vi "PXI M-Series Sync.vi"() -> ()   [LabVIEW 2012]
uses:
  <vilib>/DAQmx/write.llb/DAQmx Write (Analog 2D DBL NChan NSamp).vi
  <vilib>/DAQmx/read.llb/DAQmx Read (Digital 1D U32 1Chan NSamp).vi
  <vilib>/DAQmx/read.llb/DAQmx Read (Analog 2D I16 NChan NSamp).vi
  <vilib>/DAQmx/create/channels.llb/DAQmx Create Channel (AI-Voltage-Basic).vi
  <vilib>/DAQmx/configure/timing.llb/DAQmx Timing (Sample Clock).vi
  <vilib>/DAQmx/create/channels.llb/DAQmx Create Channel (AO-Voltage-Basic).vi
  <vilib>/DAQmx/create/channels.llb/DAQmx Create Channel (DI-Digital Input).vi
  <vilib>/DAQmx/miscellaneous.llb/DAQmx Fill In Error Info.vi
  <resource>/objmgr/daqmx.rc
panel:
  out "Trig2":bool
  out "Trig1":bool
  out "Alternative predicted rate AO":dbl
  out "RefClk.Rate":dbl
  out "SampClk.TimebaseDiv":u32
  out "SampClk.MaxRate":dbl
  in  "Desired sample rate":dbl=200000.0
  out "Predicted sample rate AI":dbl
  out "Real sample rate AI":dbl
  out "AI.Rng.Low":dbl
  out "AI.Rng.High":dbl
  out "AvailSampPerChan":u32
  out "Analog in":i16[][](graph)
  in  "stop":bool
  out "error out":errorcluster
  # "AI"
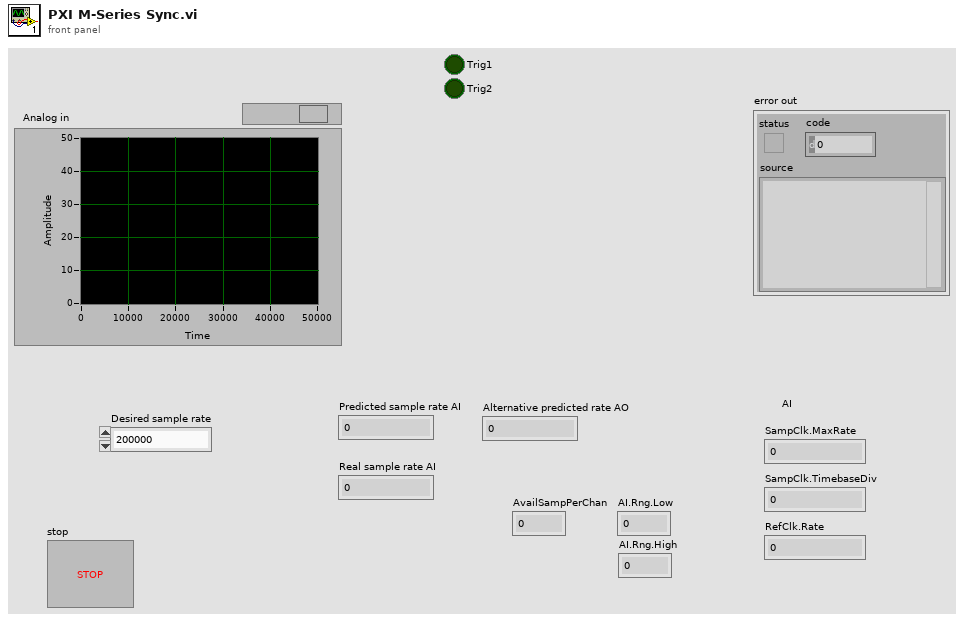
[diagram p1: front panel]
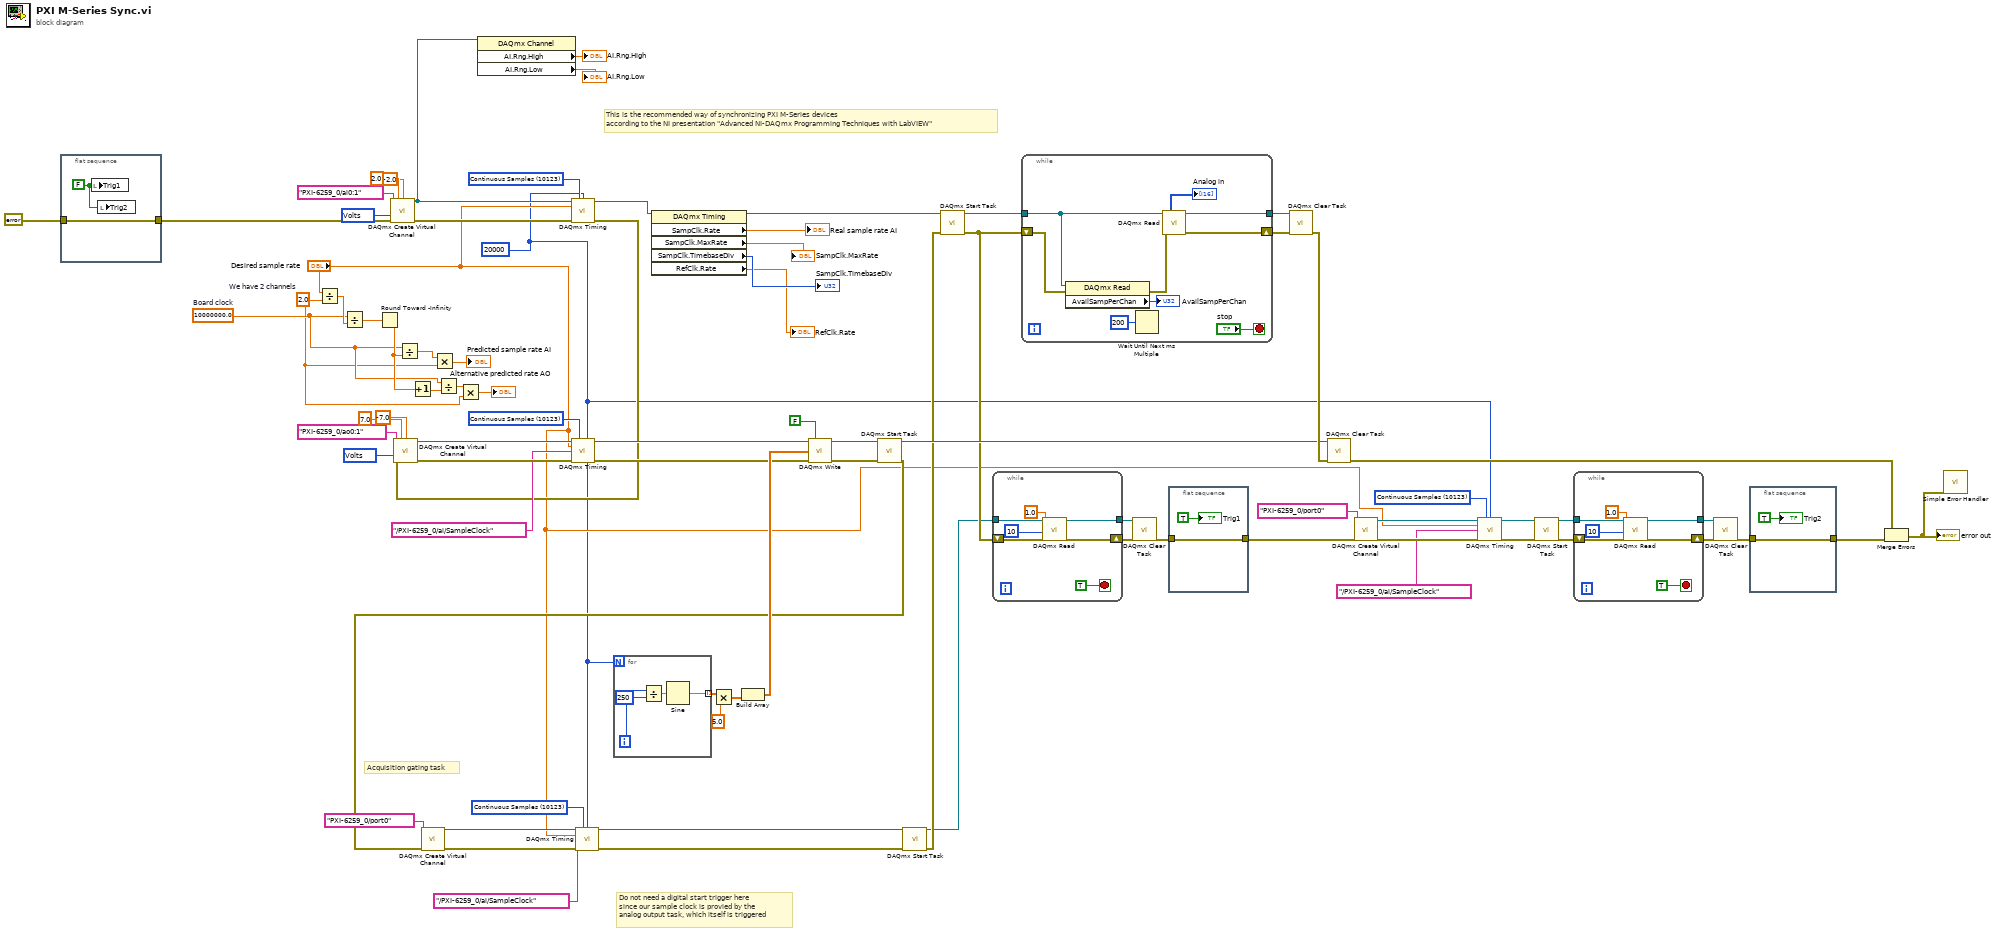
[diagram p0: block diagram]
diagram:
  w13 = 10123 items=["Finite Samples"=10178, "Continuous Samples"=10123, "Hardware Timed Single Point"=12522] ("sample mode")
  w36 = 10123 items=["Finite Samples"=10178, "Continuous Samples"=10123, "Hardware Timed Single Point"=12522] ("sample mode")
  w41 = 2.0  # We have 2 channels
  w43 = 10000000.0  # Board clock
  w62 = 10348 items=["Volts"=10348, "From Custom Scale"=10065] ("units")
  w67 = 10348 items=["Volts"=10348, "From Custom Scale"=10065] ("units")
  w78 = 10123 items=["Finite Samples"=10178, "Continuous Samples"=10123, "Hardware Timed Single Point"=12522] ("sample mode")
  w3 = 20000 ("samples per channel")
  w81 = 10123 items=["Finite Samples"=10178, "Continuous Samples"=10123, "Hardware Timed Single Point"=12522] ("sample mode")
  # "Do not need a digital start trigger here\nsince our sample clock is provied by the\nanalog output task, which itself is triggered"
  # "Acquisition gating task"
  # "This is the recommended way of synchronizing PXI M-Series devices\naccording to the NI presentation \"Advanced NI-DAQmx Programming Techniques with LabVIEW\""
  n1 = flat-sequence {
    tunnel: errorcluster {"status"=FALSE, "code"=0, "source"=""} ("error in") -> [w83]
    tunnel: [w83] -> w1
    frame #0 {
      w84 = FALSE ("Trig1")
      n2 = local write "Trig1"(w84) -> ()
      n3 = local write "Trig2"(w84) -> ()
    }
  }
  n4 = Divide(x="Desired sample rate", y=w41) -> (x/y=w48:dbl)
  n5 = Divide(x=w43, y=w48) -> (x/y=w52:dbl)
  n6 = Round Toward -Infinity(1:w52) -> (0:w45:dbl)
  n7 = call-poly <vilib>:"DAQmx Create Virtual Channel.vi"("maximum value"=2.0, "minimum value"=-2.0, "physical channels"=tag "PXI-6259_0/ai0:1", "units"=w62, "error in"=w1) -> ("task out"=w57:refnum<k21>, "error out"=w82:errorcluster)  [unwired: 9 in]
  n8 = Divide(x=w43, y=w45) -> (x/y=w47:dbl)
  n9 = Increment(x=w45) -> (x+1=w44:dbl)
  n10 = Multiply(x=w47, y=w41) -> (x*y=→"Predicted sample rate AI":dbl)
  n11 = Divide(x=w43, y=w44) -> (x/y=w42:dbl)
  n12 = Multiply(x=w42, y=w41) -> (x*y=→"Alternative predicted rate AO":dbl)
  n13 = property class="DAQmx Channel"(reference=w57) -> ("AI.Rng.High"=→"AI.Rng.High":dbl, "AI.Rng.Low"=→"AI.Rng.Low":dbl)  [unwired: 1 in, 2 out]
  n14 = call-poly <vilib>:"DAQmx Timing.vi"("task/channels in"=w57, "sample mode"=w81, "samples per channel"=w3, "rate"="Desired sample rate", "error in"=w82) -> ("task out"=w22:refnum<k21>, "error out"=w23:errorcluster)  [unwired: 9 in]
  n15 = call-poly <vilib>:"DAQmx Create Virtual Channel.vi"("maximum value"=7.0, "minimum value"=-7.0, "physical channels"=tag "PXI-6259_0/ao0:1", "units"=w67, "error in"=w23) -> ("task out"=w59:refnum<k21>, "error out"=w58:errorcluster)  [unwired: 9 in]
  n16 = call-poly <vilib>:"DAQmx Timing.vi"("task/channels in"=w59, "sample mode"=w78, "samples per channel"=w3, "rate"="Desired sample rate", "source"=tag "/PXI-6259_0/ai/SampleClock", "error in"=w58) -> ("task out"=w25:refnum<k21>, "error out"=w26:errorcluster)  [unwired: 8 in]
  n17 = for {
    N: w3 -> [_]
    tunnel: [w85] -> w69 mode=indexing
    i -> [w87]
    n18 = Divide(x=w87, y=250) -> (x/y=w88:dbl)
    n19 = Sine(x=w88) -> (sin(x)=w85:dbl)
  }
  n20 = property class="DAQmx Timing"(reference=w22) -> (reference out=w54:refnum<k21>, "SampClk.Rate"=→"Real sample rate AI":dbl, "SampClk.MaxRate"=→"SampClk.MaxRate":dbl, "SampClk.TimebaseDiv"=→"SampClk.TimebaseDiv":u32, "RefClk.Rate"=→"RefClk.Rate":dbl)  [unwired: 1 in, 1 out]
  n21 = Multiply(x=w69, y=5.0) -> (x*y=w61:dbl[])
  n22 = Build Array(w61, w61) -> (w60:dbl[][])
  n23 = call-poly <vilib>:"DAQmx Write.vi"("task/channels in"=w25, "auto start"=FALSE, "data"=w60, "error in"=w26) -> ("task out"=w77:refnum<k21>, "error out"=w75:errorcluster)  [unwired: 9 in, 1 out]
  n24 = call <vilib>:"DAQmx Start Task.vi"("task/channels in"=w77, "error in"=w75) -> ("task out"=w70:refnum<k21>, "error out"=w35:errorcluster)  [unwired: 12 in]
  n25 = call-poly <vilib>:"DAQmx Create Virtual Channel.vi"("lines"=tag "PXI-6259_0/port0", "error in"=w35) -> ("task out"=w37:refnum<k21>, "error out"=w38:errorcluster)  [unwired: 12 in]
  n26 = call-poly <vilib>:"DAQmx Timing.vi"("task/channels in"=w37, "sample mode"=w36, "samples per channel"=w3, "rate"="Desired sample rate", "source"=tag "/PXI-6259_0/ai/SampleClock", "error in"=w38) -> ("task out"=w28:refnum<k21>, "error out"=w27:errorcluster)  [unwired: 8 in]
  n27 = call <vilib>:"DAQmx Start Task.vi"("task/channels in"=w28, "error in"=w27) -> ("task out"=w31:refnum<k21>, "error out"=w34:errorcluster)  [unwired: 12 in]
  n28 = call <vilib>:"DAQmx Start Task.vi"("task/channels in"=w54, "error in"=w34) -> ("task out"=w74:refnum<k21>, "error out"=w32:errorcluster)  [unwired: 12 in]
  n29 = while {
    tunnel: w31 -> [w94]
    shift-right: [w92] -> w20
    shift-left: w32 -> [w93]
    tunnel: [w90] -> w21
    stop <- TRUE stop-if-true
    n30 = call-poly <vilib>:"DAQmx Read.vi"("task/channels in"=w94, "number of samples per channel"=10, "timeout"=1.0, "error in"=w93) -> ("task out"=w90:refnum<k21>, "error out"=w92:errorcluster)  [unwired: 9 in, 1 out]
  }
  n31 = while {
    tunnel: w74 -> [w100]
    shift-right: [w103] -> w73
    shift-left: w32 -> [w98]
    tunnel: [w102] -> w72
    stop <- "stop" stop-if-true
    n32 = property class="DAQmx Read"(reference=w100, error in=w98) -> (error out=w97:errorcluster, "AvailSampPerChan"=→"AvailSampPerChan":u32)  [unwired: 1 out]
    n33 = Wait Until Next ms Multiple(millisecond multiple=u32 200) -> ()  [unwired: 1 out]
    n34 = call-poly <vilib>:"DAQmx Read.vi"("task/channels in"=w100, "error in"=w97) -> ("task out"=w102:refnum<k21>, "data"=→"Analog in":i16[][], "error out"=w103:errorcluster)  [unwired: 11 in]
  }
  n35 = call <vilib>:"DAQmx Clear Task.vi"("task in"=w21, "error in"=w20) -> ("error out"=w19:errorcluster)  [unwired: 13 in]
  n36 = flat-sequence {
    tunnel: w19 -> [w105]
    tunnel: [w105] -> w17
    frame #0 {
      "Trig1" <- TRUE ("Trig1")
    }
  }
  n37 = call <vilib>:"DAQmx Clear Task.vi"("task in"=w72, "error in"=w73) -> ("error out"=w71:errorcluster)  [unwired: 13 in]
  n38 = call <vilib>:"DAQmx Clear Task.vi"("task in"=w70, "error in"=w71) -> ("error out"=w30:errorcluster)  [unwired: 13 in]
  n39 = call-poly <vilib>:"DAQmx Create Virtual Channel.vi"("lines"=tag "PXI-6259_0/port0", "error in"=w17) -> ("task out"=w16:refnum<k21>, "error out"=w15:errorcluster)  [unwired: 12 in]
  n40 = call-poly <vilib>:"DAQmx Timing.vi"("task/channels in"=w16, "sample mode"=w13, "samples per channel"=w3, "rate"="Desired sample rate", "source"=tag "/PXI-6259_0/ai/SampleClock", "error in"=w15) -> ("task out"=w11:refnum<k21>, "error out"=w12:errorcluster)  [unwired: 8 in]
  n41 = call <vilib>:"DAQmx Start Task.vi"("task/channels in"=w11, "error in"=w12) -> ("task out"=w6:refnum<k21>, "error out"=w7:errorcluster)  [unwired: 12 in]
  n42 = while {
    tunnel: w6 -> [w112]
    shift-right: [w110] -> w9
    shift-left: w7 -> [w111]
    tunnel: [w108] -> w10
    stop <- TRUE stop-if-true
    n43 = call-poly <vilib>:"DAQmx Read.vi"("task/channels in"=w112, "number of samples per channel"=10, "timeout"=1.0, "error in"=w111) -> ("task out"=w108:refnum<k21>, "error out"=w110:errorcluster)  [unwired: 9 in, 1 out]
  }
  n44 = call <vilib>:"DAQmx Clear Task.vi"("task in"=w10, "error in"=w9) -> ("error out"=w8:errorcluster)  [unwired: 13 in]
  n45 = flat-sequence {
    tunnel: w8 -> [w114]
    tunnel: [w114] -> w5
    frame #0 {
      "Trig2" <- TRUE ("Trig1")
    }
  }
  n46 = Merge Errors(w30, w5) -> (w29:errorcluster)
  "error out" <- w29
  n47 = call <vilib>:"Simple Error Handler.vi"("error in (no error)"=w29) -> ()  [unwired: 4 in, 5 out]
